vi "DWF MSO Query Trigger Type.vi"(0 "Instrument Handle In":u32, 11 "Error In":errorcluster caption="Error In (no error)", 12 "Trigger Instance":i32(ring) caption="Trigger Instance (A)" items=["A", "B"]) -> (4 "Instrument Handle Out":u32, 6 "Trigger Type":i32(ring) items=["Immediate", "Analog Edge", "Digital Edge", "Digital Pattern", "Digital Glitch"], 15 "Error Out":errorcluster)   [LabVIEW 2015, in "DigilentWF.lvlib"]
doc: "Indicates the trigger type of the specified instance."
uses:
  <vilib>/DigilentWF/DigilentWF.lvlib
  dwf.dll
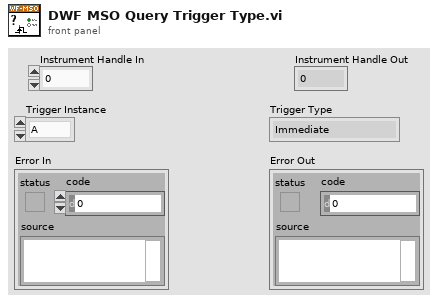
[diagram p1: front panel]
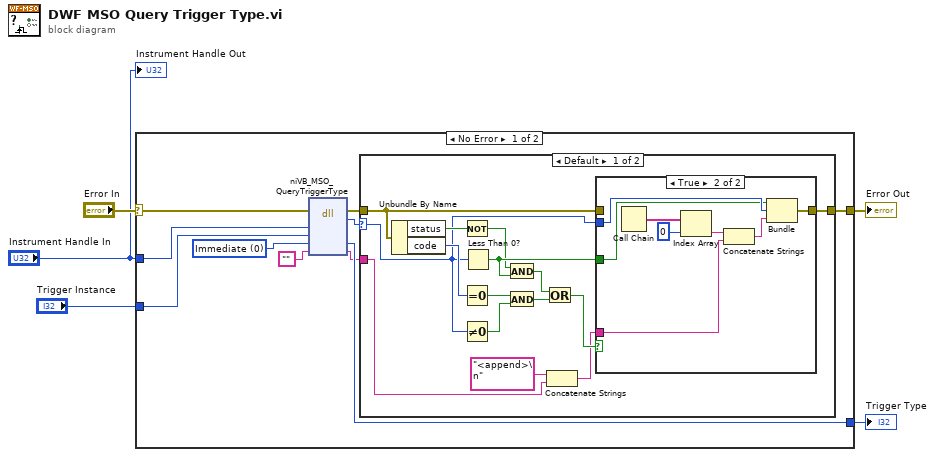
[diagram p0: block diagram]
diagram:
  n1 = case "outter_case" shown="No Error" "Error In" {
    selector: "Error In" -> [w15 w41]
    tunnel: [w12 w41] -> w4
    tunnel: "Instrument Handle In" -> [w11 _]
    tunnel: "Trigger Instance" -> [w10 _]
    tunnel: [w8 _] -> w1
    frame No Error {
      w9 = 0 items=["Immediate", "Analog Edge", "Digital Edge", "Digital Pattern", "Digital Glitch"] ("Trigger Type")
      n2 = dll-call lib="dwf.*" fn="niVB_MSO_QueryTriggerType"(error in=w15, "InstrumentHandle"=w11, "TriggerInstance"=w10, "TriggerType"=w9, "szError"="") -> (error out=w14:errorcluster, "return type"=w13:i32, "TriggerType"=w8:i32, "szError"=w6:string)  [unwired: 4 in, 1 out]
      n3 = case "inner_case" shown="Default" w13 {
        selector: w13 -> [w20 _]
        tunnel: w14 -> [w21 w40]
        tunnel: [w17 w40] -> w12
        tunnel: w6 -> [w16 _]
        frame Default {
          n4 = Unbundle By Name(w21) -> ("status"=w25:bool, "code"=w29:i32)
          n5 = Not(x=w25) -> (.not. x?=w28:bool)
          n6 = Equal To 0?(x=w29) -> (x = 0?=w24:bool)
          n7 = Not Equal To 0?(x=w20) -> (x != 0?=w27:bool)
          n8 = Less Than 0?(x=w20) -> (x < 0?=w30:bool)
          n9 = And(x=w28, y=w30) -> (x .and. y?=w26:bool)
          n10 = And(x=w24, y=w27) -> (x .and. y?=w23:bool)
          n11 = Or(x=w26, y=w23) -> (x .or. y?=w22:bool)
          n12 = Concatenate Strings("<append>\n" ("string"), w16) -> (w19:string)
          n13 = case shown="True" w22 {
            tunnel: [w31 w38] -> w17
            tunnel: w20 -> [_ w37]
            tunnel: w30 -> [_ w36]
            tunnel: w21 -> [w31 _]
            tunnel: w19 -> [_ w32]
            frame False {
            }
            frame True {
              n14 = Call Chain() -> (call chain=w35:string[])
              n15 = Index Array(array=w35, index=0) -> (element=w34:string)
              n16 = Concatenate Strings(w34, w32) -> (w39:string)
              n17 = Bundle(w36, "return type"=w37, w39) -> (w38:cluster{bool, "return type":i32, string})  [unwired: 1 out]
            }
          }
        }
        frame 0 {
        }
      }
    }
    frame Error {
    }
  }
  "Error Out" <- w4
  "Trigger Type" <- w1
  "Instrument Handle Out" <- "Instrument Handle In"
